vi "Passing Paramters Array Of Integers.vi"(8 "error in (no error)":errorcluster, 10 "length":i32, 11 "x":i32[](array[numeric])=array[4097 elements]) -> (0 "error out":errorcluster, 2 "function return":i32, 3 "x out":i32[](array[numeric]))   [LabVIEW 2009, in "LabVIEWWrapper_PassingDataSampleDLL.lvlib"]
doc: "int PassingParamters_ArrayOfIntegers (int x[], int length);"
uses:
  LabVIEWWrapper_PassingDataSampleDLL.lvlib
  PassingDataSampleDLL.dll
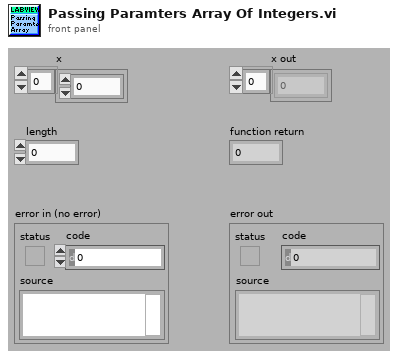
[diagram p1: front panel]
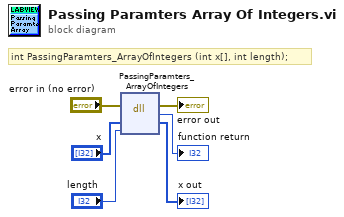
[diagram p0: block diagram]
diagram:
  # "int PassingParamters_ArrayOfIntegers (int x[], int length);"
  n1 = dll-call lib="C:/My Dropbox/Systems Engineering Application/SDK/C Integration/LabVIEWWrapper/PassingDataSampleDLL.*" fn="PassingParamters_ArrayOfIntegers"(error in="error in (no error)", "x"="x", "length"="length") -> (error out=→"error out":errorcluster, →"function return":i32, "x"=→"x out":i32[])  [unwired: 3 in, 1 out]
